vi "add-or-increment.vi"(6 "tool# or drive subsystem name":string, 9 "Position if found":i32, 10 "Found?":bool, 11 "Tool array in":T1[](array[typedef])) -> (3 "Tool array out":T1[](array[typedef]))   [LabVIEW 2017, in "labview-standard-library.lvlib" / "automode-scripting.lvlib"]
uses:
  automode-scripting.lvlib
  type-defs/tool-call-tracker.ctl
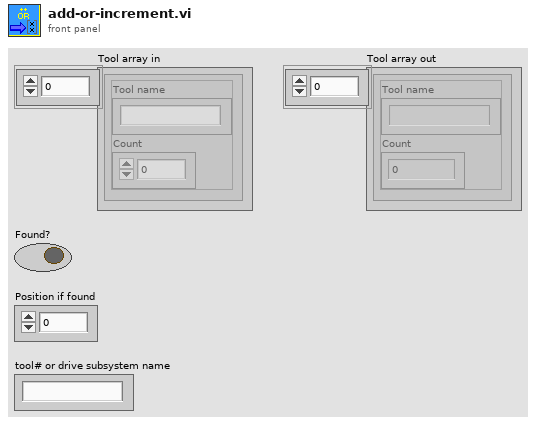
[diagram p1: front panel]
types:
  T1 = typedef "tool-call-tracker.ctl" = cluster{"Tool name":string, "Count":i32}
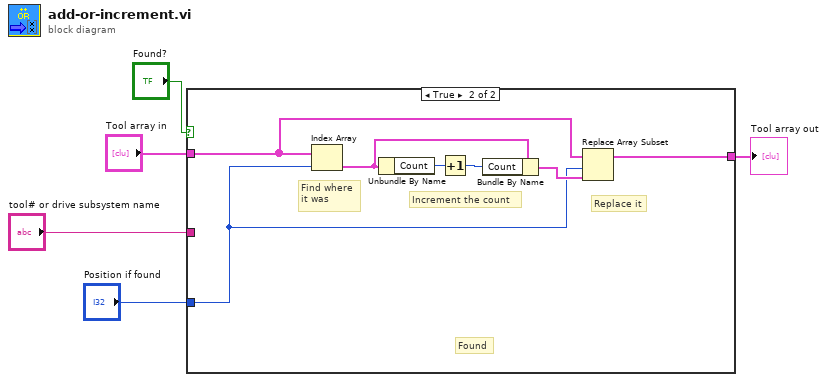
[diagram p0: block diagram]
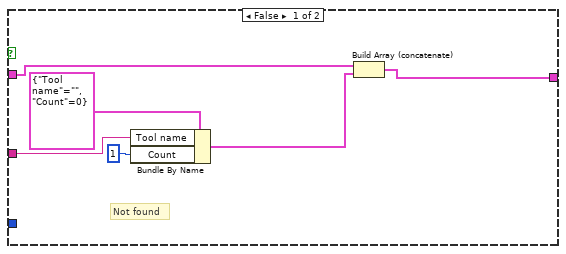
[diagram p2: hidden frame]
diagram:
  n1 = case shown="True" "Found?" {
    tunnel: "Tool array in" -> [w8 w15]
    tunnel: "tool# or drive subsystem name" -> [w10 _]
    tunnel: "Position if found" -> [_ w13]
    tunnel: [w6 w12] -> w5
    frame False {
      # "Not found"
      n2 = Bundle By Name(cluster=T1 {"Tool name"="", "Count"=0}, "Tool name"=w10, "Count"=1) -> (w7:T1)
      n3 = Build Array (concatenate)(w8, w7) -> (w6:T1[])
    }
    frame True {
      # "Replace it"
      # "Increment the count"
      # "Find where\nit was"
      # "Found"
      n4 = Index Array(array=w15, index=w13) -> (element=w17:T1)
      n5 = Unbundle By Name(w17) -> ("Count"=w18:i32)
      n6 = Increment(x=w18) -> (x+1=w16:i32)
      n7 = Bundle By Name(cluster=w17, "Count"=w16) -> (w14:T1)
      n8 = Replace Array Subset(array=w15, new element=w14, index=w13) -> (w12:T1[])
    }
  }
  "Tool array out" <- w5
